vi "Overflow buffer.vi"() -> ()   [LabVIEW 2021]
uses:
  <vilib>/DAQmx/write.llb/DAQmx Write (Analog DBL 1Chan 1Samp).vi
  <vilib>/DAQmx/read.llb/DAQmx Read (Analog 1D DBL 1Chan NSamp).vi
  <vilib>/DAQmx/create/channels.llb/DAQmx Create Channel (AI-Voltage-Basic).vi
  <vilib>/DAQmx/configure/timing.llb/DAQmx Timing (Sample Clock).vi
  <vilib>/DAQmx/miscellaneous.llb/DAQmx Fill In Error Info.vi
  <vilib>/DAQmx/create/channels.llb/DAQmx Create Channel (AO-Voltage-Basic).vi
panel:
  in  "Slide":dbl(slide) scale=-5.0..5.0
  in  "milliseconds to wait":u32
  in  "stop 2":bool
  out "Waveform Chart":dbl[](graph)
  in  "stop":bool
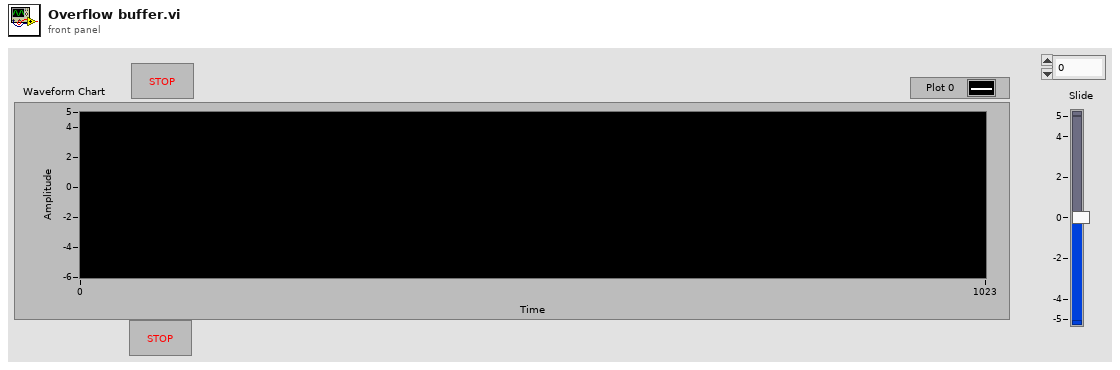
[diagram p1: front panel]
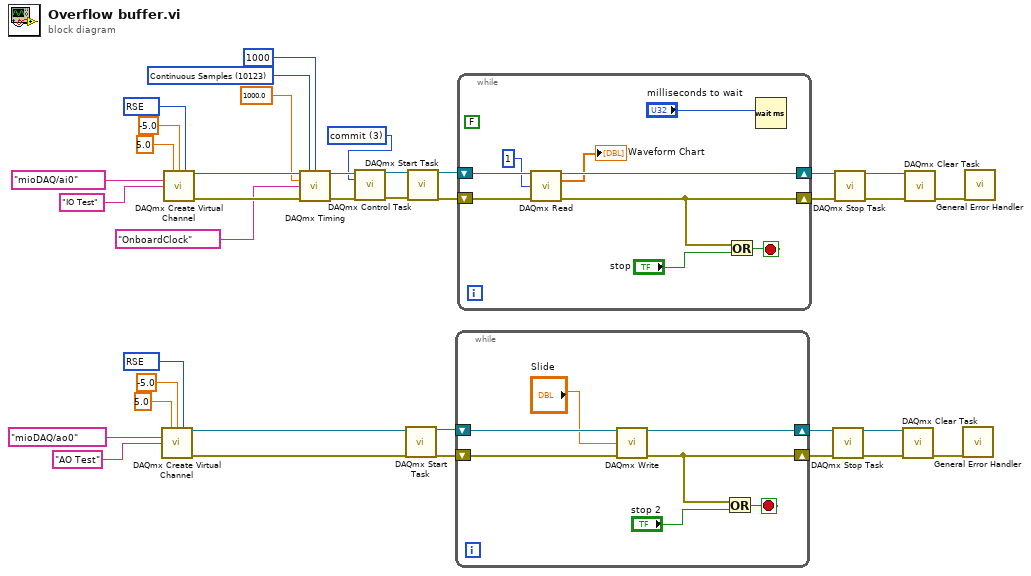
[diagram p0: block diagram]
diagram:
  w1 = 10083 items=["Default"=-1, "RSE"=10083, "Differential"=10106, "Pseudodifferential"=12529] ("output terminal configuration")
  w2 = 10083 items=["Default"=-1, "RSE"=10083, "NRSE"=10078, "Differential"=10106, "Pseudodifferential"=12529] ("input terminal configuration")
  w18 = 3 items=["verify"=2, "reserve"=4, "commit"=3, "unreserve"=5, "abort"=6] ("action")
  w30 = 10123 items=["Finite Samples"=10178, "Continuous Samples"=10123, "Hardware Timed Single Point"=12522] ("sample mode")
  n1 = call-poly <vilib>:"DAQmx Create Virtual Channel.vi"("maximum value"=5.0, "minimum value"=-5.0, "output terminal configuration"=w1, "physical channels"=tag "mioDAQ/ao0", "name to assign"="AO Test") -> ("task out"=w4:refnum<k21>, "error out"=w5:errorcluster)  [unwired: 9 in]
  n2 = call-poly <vilib>:"DAQmx Create Virtual Channel.vi"("maximum value"=5.0, "minimum value"=-5.0, "input terminal configuration"=w2, "physical channels"=tag "mioDAQ/ai0", "name to assign"="IO Test") -> ("task out"=w37:refnum<k21>, "error out"=w36:errorcluster)  [unwired: 9 in]
  n3 = call-poly <vilib>:"DAQmx Timing.vi"("task/channels in"=w37, "sample mode"=w30, "samples per channel"=1000, "rate"=1000.0, "source"=tag "OnboardClock", "error in"=w36) -> ("task out"=w22:refnum<k21>, "error out"=w21:errorcluster)  [unwired: 8 in]
  n4 = call <vilib>:"DAQmx Control Task.vi"("task/channels in"=w22, "action"=w18, "error in"=w21) -> ("task out"=w20:refnum<k21>, "error out"=w19:errorcluster)  [unwired: 11 in]
  n5 = call <vilib>:"DAQmx Start Task.vi"("task/channels in"=w4, "error in"=w5) -> ("task out"=w14:refnum<k21>, "error out"=w15:errorcluster)  [unwired: 12 in]
  n6 = call <vilib>:"DAQmx Start Task.vi"("task/channels in"=w20, "error in"=w19) -> ("task out"=w17:refnum<k21>, "error out"=w16:errorcluster)  [unwired: 12 in]
  n7 = while {
    shift-right: [w42] -> w6
    shift-left: w14 -> [w44]
    shift-right: [w40] -> w7
    shift-left: w15 -> [w43]
    stop <- w39 stop-if-true
    n8 = call-poly <vilib>:"DAQmx Write.vi"("task/channels in"=w44, "data"="Slide", "error in"=w43) -> ("task out"=w42:refnum<k21>, "error out"=w40:errorcluster)  [unwired: 10 in, 1 out]
    n9 = Or(x=w40, y="stop 2") -> (x .or. y?=w39:bool)
  }
  n10 = while {
    shift-right: [w51] -> w35
    shift-left: w17 -> [w53]
    shift-right: [w49] -> w34
    shift-left: w16 -> [w52]
    stop <- w48 stop-if-true
    (unwired) FALSE
    n11 = call-poly <vilib>:"DAQmx Read.vi"("task/channels in"=w53, "number of samples per channel"=1, "error in"=w52) -> ("task out"=w51:refnum<k21>, "data"=→"Waveform Chart":dbl[], "error out"=w49:errorcluster)  [unwired: 10 in]
    n12 = Or(x=w49, y="stop") -> (x .or. y?=w48:bool)
    n13 = Wait (ms)(milliseconds to wait="milliseconds to wait") -> ()  [unwired: 1 out]
  }
  n14 = call <vilib>:"DAQmx Stop Task.vi"("task/channels in"=w6, "error in"=w7) -> ("task out"=w8:refnum<k21>, "error out"=w9:errorcluster)  [unwired: 12 in]
  n15 = call <vilib>:"DAQmx Stop Task.vi"("task/channels in"=w35, "error in"=w34) -> ("task out"=w33:refnum<k21>, "error out"=w32:errorcluster)  [unwired: 12 in]
  n16 = call <vilib>:"DAQmx Clear Task.vi"("task in"=w8, "error in"=w9) -> ("error out"=w10:errorcluster)  [unwired: 13 in]
  n17 = call <vilib>:"DAQmx Clear Task.vi"("task in"=w33, "error in"=w32) -> ("error out"=w31:errorcluster)  [unwired: 13 in]
  n18 = call <vilib>:"General Error Handler.vi"("error in (no error)"=w10) -> ()  [unwired: 10 in, 5 out]
  n19 = call <vilib>:"General Error Handler.vi"("error in (no error)"=w31) -> ()  [unwired: 10 in, 5 out]
